vi "Write All Pending Data.vi"(8 "error in (no error)":errorcluster, 9 "byte order":T1(ring)=enum."little-endian", 10 "Pending data":refnum<data-value>[](array[refnum]), 11 "refnum in":refnum<file>) -> (0 "error out":errorcluster, 3 "refnum out":refnum<file>)   [LabVIEW 2016]
uses:
  Tag/Offset Content.ctl
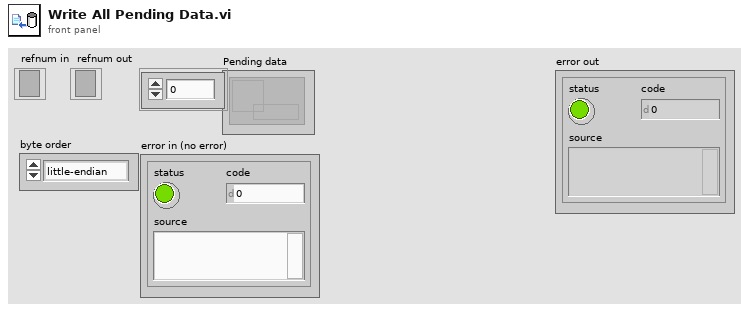
[diagram p1: front panel]
types:
  T1 = enum16{"big-endian, network order", "native, host order", "little-endian"}
  T2 = typedef "Offset Content.ctl" = cluster{"Pointer Byte Offset":u32, "Content":string}
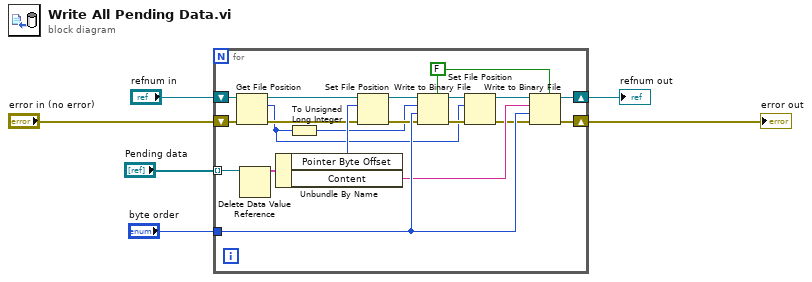
[diagram p0: block diagram]
diagram:
  n1 = for {
    shift-right: [w16] -> w3
    shift-left: "refnum in" -> [w24]
    tunnel: "Pending data" -> [w26] mode=indexing
    tunnel: "byte order" -> [w18]
    shift-right: [w10] -> w1
    shift-left: "error in (no error)" -> [w15]
    w9 = FALSE ("prepend array or string size? (T)")
    n2 = Get File Position(4:w15, 7:w24) -> (0:w14:errorcluster, 2:w7:i64, 3:w20:refnum<file>)
    n3 = Delete Data Value Reference(data value reference=w26) -> (data value=w25:T2)  [unwired: 1 in, 1 out]
    n4 = Unbundle By Name(w25) -> ("Pointer Byte Offset"=w23:u32, "Content"=w17:string)
    n5 = To Unsigned Long Integer(number=w7) -> (unsigned 32bit integer=w8:u32)
    n6 = Set File Position(offset (in bytes) (0)=w23, refnum=w20, error in=w14) -> (refnum out=w22:refnum<file>, error out=w13:errorcluster)  [unwired: 1 in]
    n7 = Write to Binary File(file (use dialog)=w22, data=w8, error in=w13, 5:w9, 9:w18) -> (refnum out=w21:refnum<file>, error out=w12:errorcluster)  [unwired: 1 in, 1 out]
    n8 = Set File Position(offset (in bytes) (0)=w7, refnum=w21, error in=w12) -> (refnum out=w19:refnum<file>, error out=w11:errorcluster)  [unwired: 1 in]
    n9 = Write to Binary File(file (use dialog)=w19, data=w17, error in=w11, 5:w9, 9:w18) -> (refnum out=w16:refnum<file>, error out=w10:errorcluster)  [unwired: 1 in, 1 out]
  }
  "refnum out" <- w3
  "error out" <- w1
